vi "Start Sync.vi"(8 "error in (no error)":errorcluster, 11 "gRPC Server in":refnum<class "WaveformMonitor.lvclass">) -> (0 "error out":errorcluster, 3 "gRPC Server out":refnum<class "WaveformMonitor.lvclass">)   [LabVIEW 2021, in "CIFWaveformMonitor_server.lvlib" / "WaveformMonitor.lvclass"]
uses:
  WaveformMonitor.lvclass
  WaveformMonitor.lvclass/WaveformMonitor.ctl
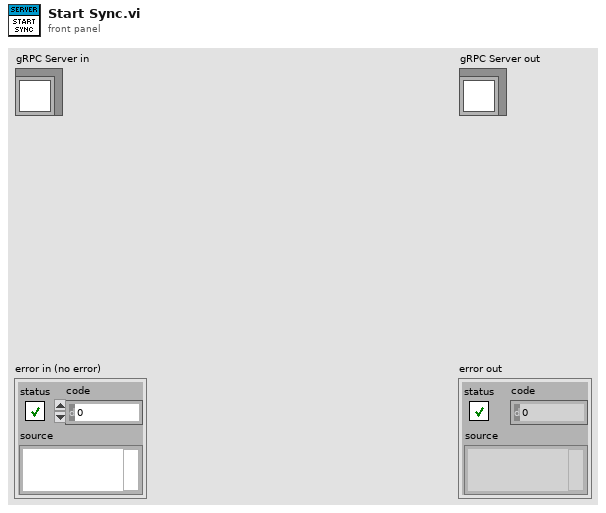
[diagram p1: front panel]
types:
  T1 = typedef "CIFWaveformMonitor_server.lvlib/WaveformMonitor.lvclass/Server Internal UEs.ctl" = cluster{"WaveformMonitor SetEnableWaveform Internal UE":refnum<user-event>, "WaveformMonitor GetWaveform Internal UE":refnum<user-event>}
  T2 = typedef "CIFWaveformMonitor_server.lvlib/WaveformMonitor.lvclass/Server gRPC UEs.ctl" = cluster{"WaveformMonitor SetEnableWaveform gRPC UE":refnum<user-event>, "WaveformMonitor GetWaveform gRPC UE":refnum<user-event>}
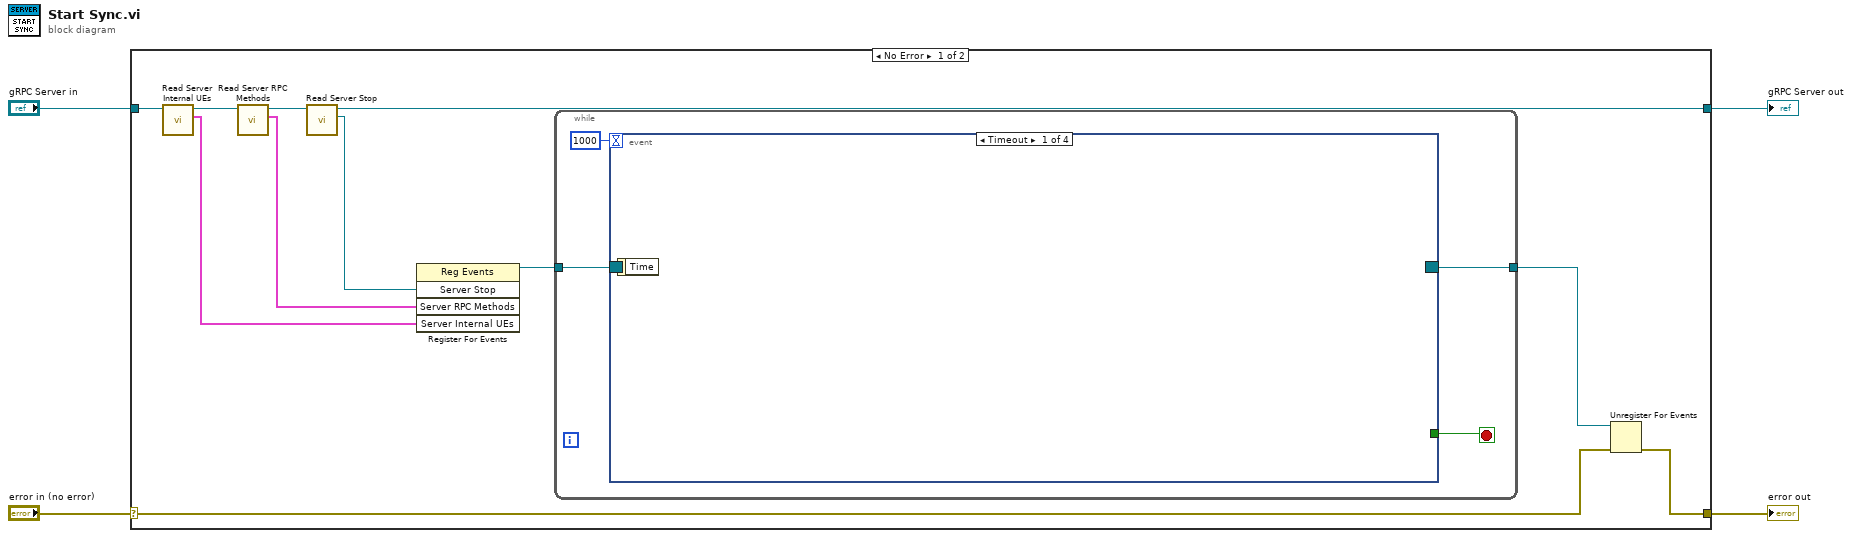
[diagram p0: block diagram]
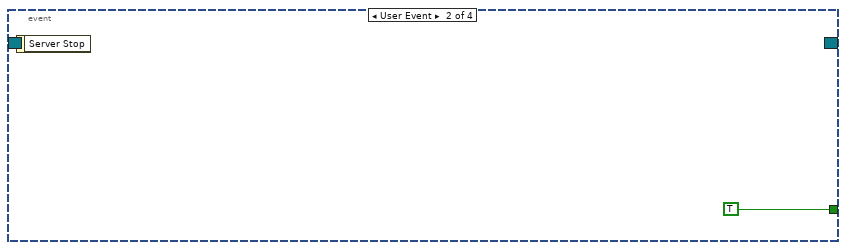
[diagram p2: hidden frame]
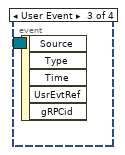
[diagram p3: hidden frame]
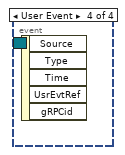
[diagram p4: hidden frame]
diagram:
  n1 = case shown="No Error" "error in (no error)" {
    selector: "error in (no error)" -> [w9 w22]
    tunnel: [w8 w22] -> w3
    tunnel: [w6 w21] -> w1
    tunnel: "gRPC Server in" -> [w15 w21]
    frame No Error {
      n2 = call "Read Server Internal UEs.vi"("SignalGeneratorService in"=w15) -> ("Server Internal UEs"=w13:T1, "SignalGeneratorService out"=w14:refnum<class "WaveformMonitor.lvclass">)  [unwired: 8 in, 1 out]
      n3 = call "Read Server RPC Methods.vi"("SignalGeneratorService in"=w14) -> ("Server RPC Methods"=w7:T2, "SignalGeneratorService out"=w12:refnum<class "WaveformMonitor.lvclass">)  [unwired: 8 in, 1 out]
      n4 = call-dynamic "Read Server Stop.vi"("iService in"=w12) -> ("Server Stop"=w5:refnum<user-event>, "iService out"=w6:refnum<class "WaveformMonitor.lvclass">)  [unwired: 8 in, 1 out]
      n5 = register-events(w5, w7, w13) -> (reference out=w11:refnum<event-registration>)  [unwired: 2 in, 1 out]
      n6 = while {
        tunnel: w11 -> [w19]
        tunnel: [w17] -> w10
        stop <- w18 stop-if-true
        n7 = event "RPC Methods Event Structure" shown="[0] Timeout" {
          selector: w19 -> [_ _ _ _]
          dyn-events: [_ _ _ _] -> w17
          timeout: 1000 -> [_ _ _ _]
          tunnel: [_ TRUE _ _] -> w18
          event Timeout {
            n8 = event-data() -> ()  [unwired: 1 in, 1 out]
          }
          event User Event {
            n9 = event-data() -> ()  [unwired: 1 in, 1 out]
          }
          event User Event {
            n10 = event-data() -> ()  [unwired: 1 in, 5 out]
          }
          event User Event {
            n11 = event-data() -> ()  [unwired: 1 in, 5 out]
          }
        }
      }
      n12 = Unregister For Events(event registration refnum=w10, error in=w9) -> (error out=w8:errorcluster)
    }
    frame Error {
    }
  }
  "error out" <- w3
  "gRPC Server out" <- w1
